vi "Release Network.vi"(0 "Neural Network":T1={"Weigths"=[], "Last Layer Linear"=TRUE, "Add Bias Inputs"=TRUE, "# Inputs"=0, "# Output Neurons/Outputs"=0, "Inputs Scaling"={"X Scaling Vector"=[], "Y Scaling Vector"=[]}, "Outputs Scaling"={"X Scaling Vector"=[], "Y Scaling Vector"=[]}}, 11 "Error In":errorcluster) -> (15 "Error Out":errorcluster)   [LabVIEW 2011, in "Super Simple Neural Network.lvlib"]
doc: "This VI releases the used neural network. This does not mean anything for now and this VI is empty but it might do something more in the future."
uses:
  Super Simple Neural Network.lvlib
  Types/2D Array.ctl
  Types/Scaling Info.ctl
  Types/Neural Network.ctl
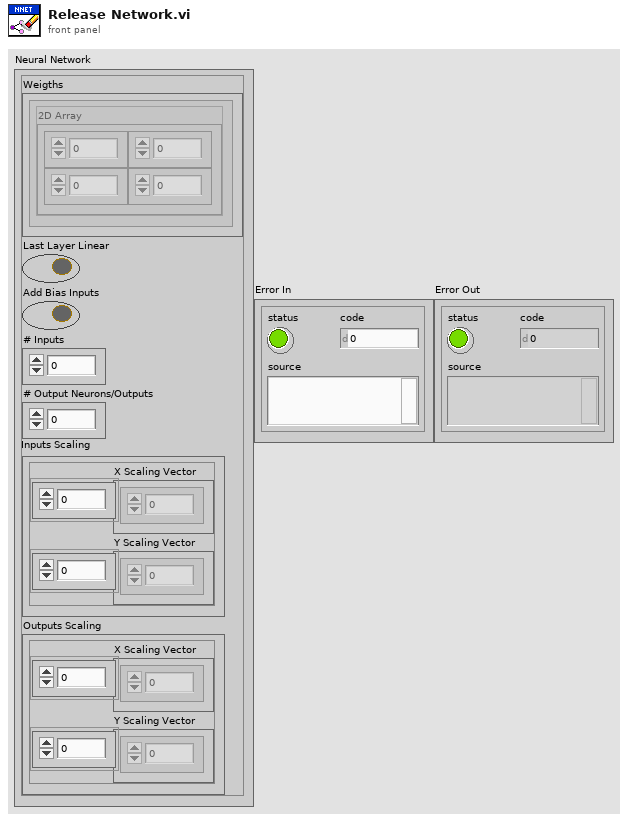
[diagram p1: front panel]
types:
  T1 = typedef "Super Simple Neural Network.lvlib/Neural Network.ctl" = cluster{"Weigths":T2[], "Last Layer Linear":bool, "Add Bias Inputs":bool, "# Inputs":u32, "# Output Neurons/Outputs":u32, "Inputs Scaling":T3, "Outputs Scaling":T3}
  T2 = typedef "Super Simple Neural Network.lvlib/2D Array.ctl" = cluster{"2D Array":dbl[][]}
  T3 = typedef "Super Simple Neural Network.lvlib/Scaling Info.ctl" = cluster{"X Scaling Vector":dbl[], "Y Scaling Vector":dbl[]}
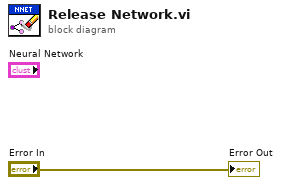
[diagram p0: block diagram]
diagram:
  "Error Out" <- "Error In"
